vi "atten_control.vi"() -> ()   [LabVIEW 2020]
uses:
  <vilib>/Instr/_visa.llb/VISA Configure Serial Port (Instr).vi
panel:
  in  "Set Rotation Speed (deg/sec)":sgl=5.0
  in  "COM Port":refnum<visa-resource-name>
  in  "Clear Laser":bool
  in  "Block Laser":bool
  in  "Home Attenuator":bool
  in  "Angle":sgl
  in  "Rotate To":bool
  in  "Set Speed":bool
  in  "stop":bool
  # "Laser Attenuator Control System"
  # "Setup Instructions"
  # "Defaults"
  # "1. Select COM port\n2. Run Program\n3. Home attenuator"
  # "• Speed = 5 deg/sec\n• Current angle = 0°\n• Laser blocked"
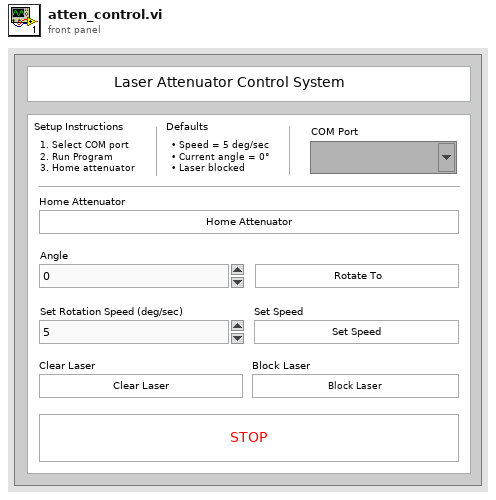
[diagram p1: front panel]
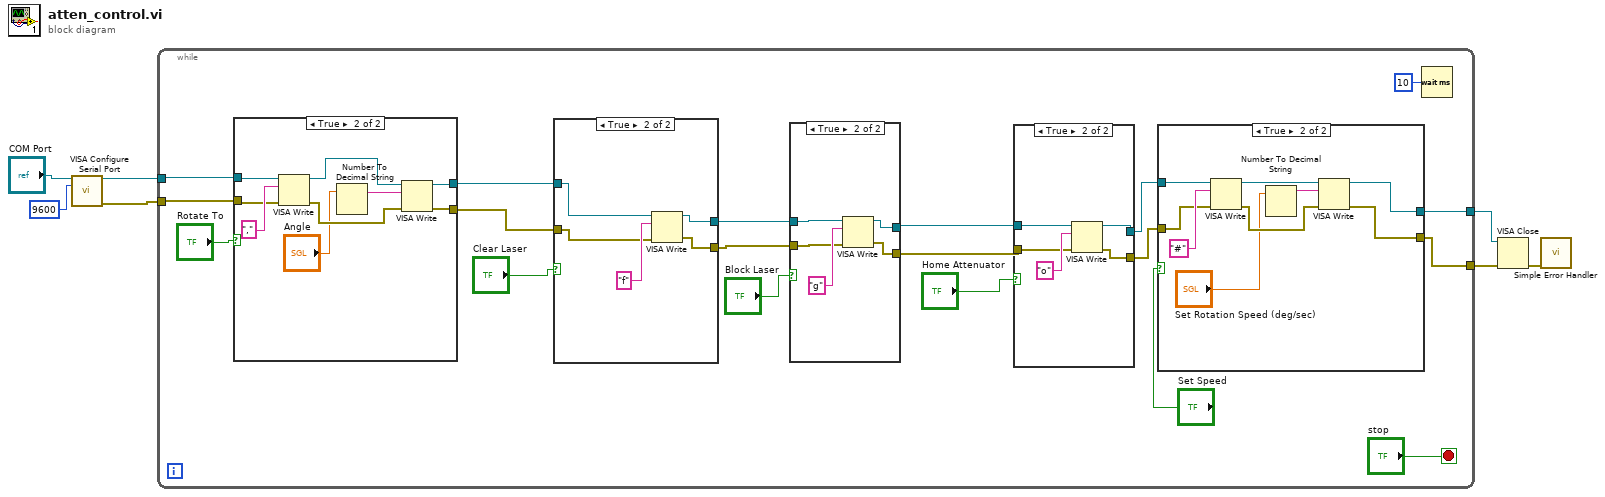
[diagram p0: block diagram]
diagram:
  n1 = call-poly "VISA Configure Serial Port"("VISA resource name"="COM Port", "baud rate (9600)"=u32 9600) -> ("VISA resource name out"=w4:refnum<visa-resource-name>, "error out"=w3:errorcluster)  [unwired: 12 in]
  n2 = while {
    tunnel: w4 -> [w12]
    tunnel: w3 -> [w11]
    tunnel: [w9] -> w2
    tunnel: [w8] -> w1
    stop <- "stop" stop-if-true
    n3 = case shown="True" "Rotate To" {
      tunnel: w12 -> [w39 w42]
      tunnel: w11 -> [w38 w41]
      tunnel: [w39 w44] -> w17
      tunnel: [w38 w43] -> w16
      frame False {
      }
      frame True {
        n4 = VISA Write(VISA resource name=w42, write buffer=",", error in (no error)=w41) -> (VISA resource name out=w47:refnum<visa-resource-name>, error out=w46:errorcluster)  [unwired: 1 out]
        n5 = Number To Decimal String(number="Angle") -> (decimal integer string=w48:string)  [unwired: 1 in]
        n6 = VISA Write(VISA resource name=w47, write buffer=w48, error in (no error)=w46) -> (VISA resource name out=w44:refnum<visa-resource-name>, error out=w43:errorcluster)  [unwired: 1 out]
      }
    }
    n7 = case shown="True" "Clear Laser" {
      tunnel: w17 -> [w64 w66]
      tunnel: w16 -> [w63 w65]
      tunnel: [w64 w68] -> w23
      tunnel: [w63 w67] -> w22
      frame False {
      }
      frame True {
        n8 = VISA Write(VISA resource name=w66, write buffer="f", error in (no error)=w65) -> (VISA resource name out=w68:refnum<visa-resource-name>, error out=w67:errorcluster)  [unwired: 1 out]
      }
    }
    n9 = case shown="True" "Block Laser" {
      tunnel: [w57 w61] -> w20
      tunnel: [w56 w60] -> w19
      tunnel: w23 -> [w57 w59]
      tunnel: w22 -> [w56 w58]
      frame False {
      }
      frame True {
        n10 = VISA Write(VISA resource name=w59, write buffer="g", error in (no error)=w58) -> (VISA resource name out=w61:refnum<visa-resource-name>, error out=w60:errorcluster)  [unwired: 1 out]
      }
    }
    n11 = case shown="True" "Home Attenuator" {
      tunnel: [w50 w52] -> w15
      tunnel: [w49 w51] -> w13
      tunnel: w20 -> [w50 w54]
      tunnel: w19 -> [w49 w53]
      frame False {
      }
      frame True {
        n12 = VISA Write(VISA resource name=w54, write buffer="o", error in (no error)=w53) -> (VISA resource name out=w52:refnum<visa-resource-name>, error out=w51:errorcluster)  [unwired: 1 out]
      }
    }
    n13 = case shown="True" "Set Speed" {
      tunnel: w15 -> [w28 w31]
      tunnel: w13 -> [w27 w30]
      tunnel: [w28 w33] -> w8
      tunnel: [w27 w32] -> w9
      frame False {
      }
      frame True {
        n14 = VISA Write(VISA resource name=w31, write buffer="#", error in (no error)=w30) -> (VISA resource name out=w36:refnum<visa-resource-name>, error out=w35:errorcluster)  [unwired: 1 out]
        n15 = Number To Decimal String(number="Set Rotation Speed (deg/sec)") -> (decimal integer string=w37:string)  [unwired: 1 in]
        n16 = VISA Write(VISA resource name=w36, write buffer=w37, error in (no error)=w35) -> (VISA resource name out=w33:refnum<visa-resource-name>, error out=w32:errorcluster)  [unwired: 1 out]
      }
    }
    n17 = Wait (ms)(milliseconds to wait=u32 10) -> ()  [unwired: 1 out]
  }
  n18 = VISA Close(VISA resource name=w1, error in (no error)=w2) -> (error out=w7:errorcluster)
  n19 = call <vilib>:"Simple Error Handler.vi"("error in (no error)"=w7) -> ()  [unwired: 4 in, 5 out]
